vi "TestStand - Read 1D Array_Numeric.vi"(0 "Sequence Context":refnum<k7>, 2 "Lookup String":string="Locals.NumericArray", 11 "Error In":errorcluster) -> (4 "Value":dbl[](array[numeric]) format="%.2f", 15 "Error Out":errorcluster)   [LabVIEW 2013]
doc: "This VI retrieves TestStand 1D Array"
uses:
  <vilib>/addons/TestStand/_TSUtility.llb/TestStand - Get Property Value (Numeric Array).vi
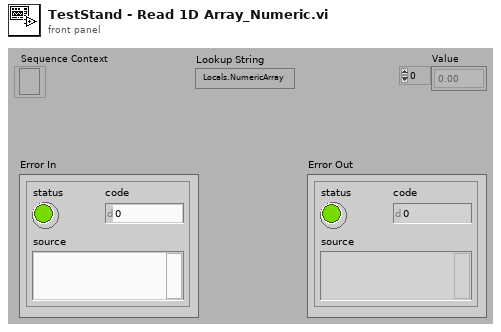
[diagram p1: front panel]
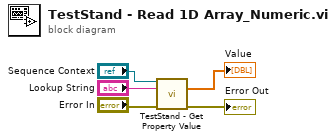
[diagram p0: block diagram]
diagram:
  n1 = call-poly <vilib>:"TestStand - Get Property Value.vi"("Sequence Context In"="Sequence Context", "Lookup String"="Lookup String", "error in (no error)"="Error In") -> ("Value"=→"Value":dbl[], "error out"=→"Error Out":errorcluster)  [unwired: 11 out]
